vi "WorkspaceOpenClose.vi"(1 "Open/Close? (T: Open)":bool) -> (0 "error out":errorcluster)   [LabVIEW 2015, in "ni-veristand-steps-runtime-lib.lvlib"]
uses:
  ni-veristand-steps-runtime-lib.lvlib
  <vilib>/NI Veristand/Execution/Project/NI_VS Project ExecutionAPI.lvlib
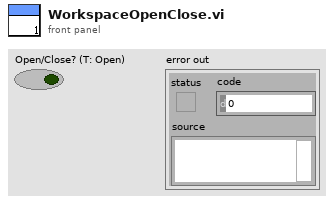
[diagram p1: front panel]
types:
  T1 = typedef "ni-veristand-steps-runtime-lib.lvlib/VeriStand dotNet References.ctl" = cluster{"ModelManager":T2, "AlarmManager":T3, "ChannelFault":T4, "WorkspaceManager":T5, "Project Ref":T6}
  T2 = typedef "NI_VS ModelManager ExecutionAPI.lvlib/ModelManagerAPI.ctl" = refnum<k24>
  T3 = typedef "NI_VS AlarmManager ExecutionAPI.lvlib/AlarmManagerAPI.ctl" = refnum<k24>
  T4 = typedef "NI_VS ChannelFault ExecutionAPI.lvlib/ChannelFaultAPI.ctl" = refnum<k24>
  T5 = typedef "NI_VS Workspace ExecutionAPI.lvlib/WorkspaceAPI.ctl" = refnum<k24>
  T6 = typedef "NI_VS Project ExecutionAPI.lvlib/Project Ref.ctl" = refnum<k24>
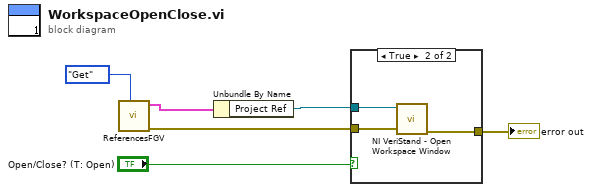
[diagram p0: block diagram]
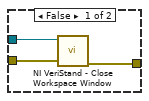
[diagram p2: hidden frame]
diagram:
  n1 = call "ReferencesFGV.vi"("Get/Set"=enum16{"Get", "Set"}."Get") -> ("error out"=w3:errorcluster, "VeriStand dotNET Refs out"=w2:T1)  [unwired: 9 in]
  n2 = Unbundle By Name(w2) -> ("Project Ref"=w1:T6)
  n3 = case shown="True" "Open/Close? (T: Open)" {
    tunnel: [w9 w12] -> w6
    tunnel: w3 -> [w8 w11]
    tunnel: w1 -> [w7 w10]
    frame False {
      n4 = call <vilib>:"NI VeriStand - Close Workspace Window.vi"("error in (no error)"=w8, "Project Ref in"=w7) -> ("error out"=w9:errorcluster)  [unwired: 8 in, 1 out]
    }
    frame True {
      n5 = call <vilib>:"NI VeriStand - Open Workspace Window.vi"("error in (no error)"=w11, "Project Ref in"=w10) -> ("error out"=w12:errorcluster)  [unwired: 8 in, 1 out]
    }
  }
  "error out" <- w6
